vi "Glavna_Programa.vi"() -> ()   [LabVIEW 2021, in "Main.lvlib"]
doc: "Main VI program. \n1. After starting the program, click PowerUP to turn on the calibrator.\n2. The program in Standby can pick the signal values with the use of the keyboard or SetUP mode. \nThe SetUP VI can configure can change the signal type, offset and phase. \n3. Click Operate to go to Operate mode. First 2 Warning message will be shown, then the program will start with Operate mode.\n4. Click Standby to go to standby again, then the program will stop with the DaQ and Operating mode.\n5. Click PowerUP to sotp the program"
uses:
  Main.lvlib
  Tipski Definicii/Kalibrator_Sostojbi.ctl
  Tipski Definicii/QMH_Daq_States.ctl
  Tipski Definicii/error_handl.ctl
  Tipski Definicii/check.ctl
  Tipski Definicii/Keyboard_Sostojbi.ctl
  Tipski Definicii/Signal Values.ctl
  Tipski Definicii/rel_error.ctl
  Tipski Definicii/danger.ctl
  Tipski Definicii/Unit.ctl
  Polymorphic/Init_Main.vi
  <vilib>/Platform/browser.llb/Open URL in Default Browser (path).vi
  Polymorphic/Enq_DaQ_QMH.vi
  Polymorphic/Enq_Calibrator_QMH.vi
  Polymorphic/Prev_Calibrator_QMH.vi
  Polymorphic/DeQ_Calibrator_QMH.vi
  Polymorphic/DaQ_Signal.vi
  Polymorphic/Release_Main.vi
  Signal/Signal.lvlib
  subVIS/Main_Programs_SubVIs.lvlib
  Polymorphic/Queues.lvlib
panel:
  out "AuxA":bool
  out "NormalV":bool
  in  "Knob":dbl(knob) scale=-3.0..3.0 scale format="%#.3g"
  out "Lev_Indikator":string
  out "Desen_Indikator":string
  out "Scope Out":bool
  out "Scope In":bool
  out "AuxAOut":bool
  out "NormalVOut":bool
  in  "V":bool
  in  "Trig":bool
  in  "Tocka":bool
  in  "0":bool
  in  "STBY":bool
  in  "Shift":bool
  in  "SetUP":bool
  in  "Scope":bool
  in  "Save":bool
  in  "Reset":bool
  in  "Power Up":bool
  in  "Plus":bool
  in  "Opr":bool
  in  "Ohm":bool
  in  "NewRef":bool
  in  "Multi":bool
  in  "Meas":bool
  in  "M":bool
  in  "k":bool
  in  "Hz":bool
  in  "F":bool
  in  "Enter":bool
  in  "Earth":bool
  in  "Div":bool
  in  "Conn?":bool
  in  "CE":bool
  in  "C":bool
  in  "Boost":bool
  in  "A":bool
  in  "9":bool
  in  "m":bool
  in  "8":bool
  in  "7":bool
  in  "6":bool
  in  "5":bool
  in  "4":bool
  in  "3":bool
  in  "2":bool
  in  "1":bool
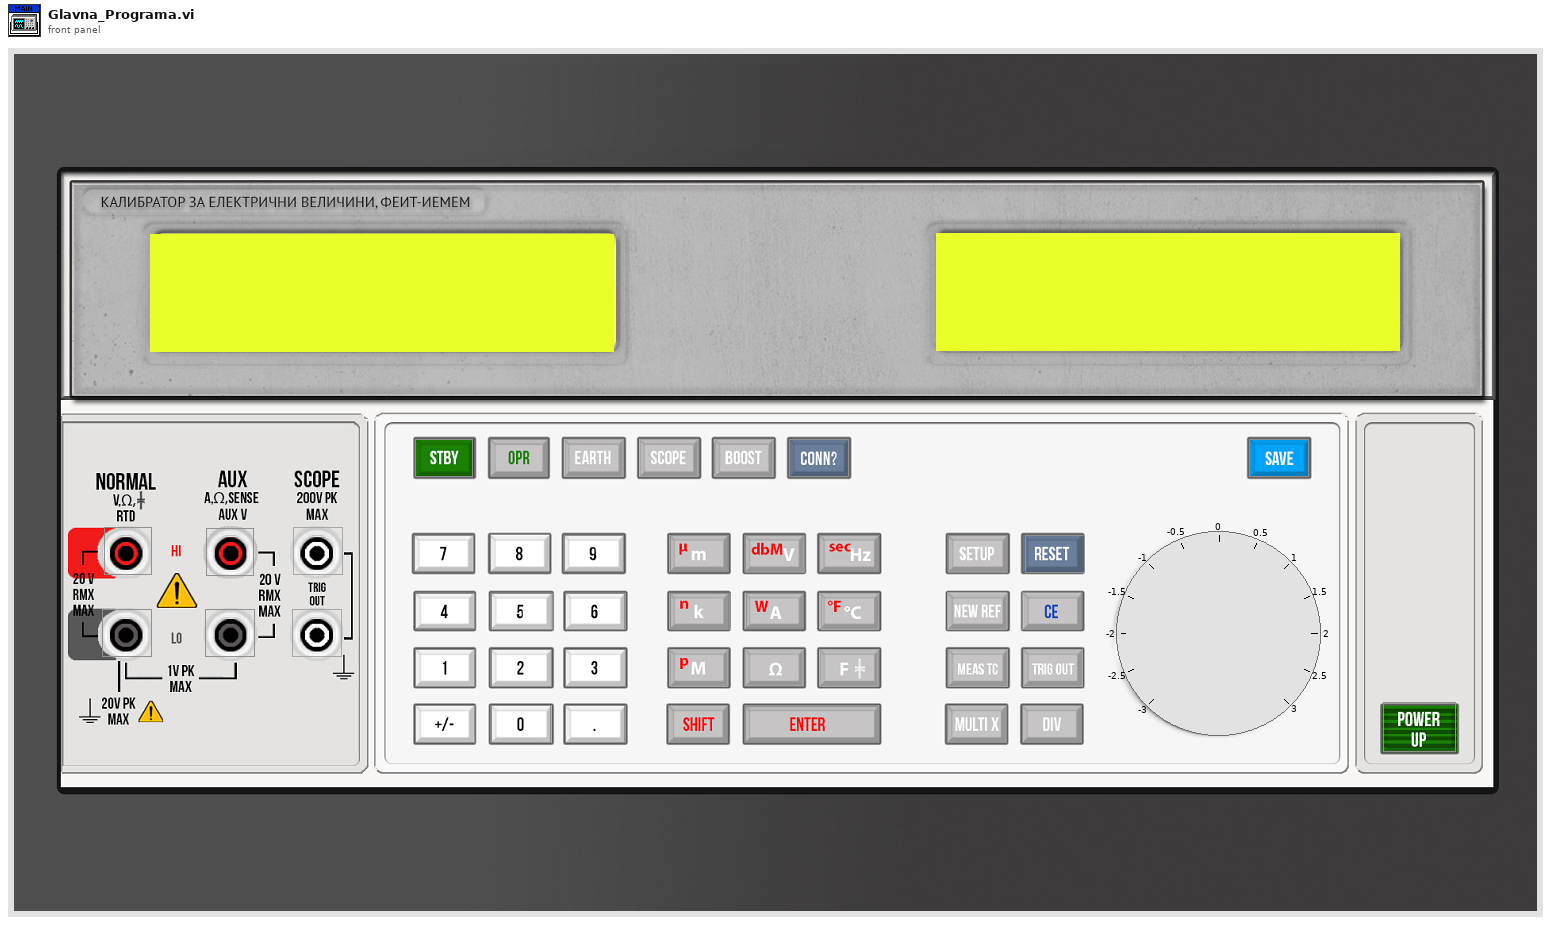
[diagram p1: front panel]
types:
  T1 = cluster{"Calibrator Queue ":refnum<queue>, "ER Refnum":refnum<event-registration>, "User Event in":refnum<user-event>, "QMH Queue ":refnum<queue>, "DaQ":refnum<queue>}
  T2 = typedef "Main_program_queues.ctl" = cluster{"Calibrator QMH":refnum<queue>, "DaQ QMH":refnum<queue>, "DaQ":refnum<queue>, "ER":refnum<event-registration>, "User Event":refnum<user-event>}
  T3 = typedef "error_handl.ctl" = enum16{"Init", "Insert Error 1", "Insert Error 2", "Insert Error 3", "Insert Error 4", "Handle Erros"}
  T4 = enum16{"Init", "Init DaQ", "Start", "Output", "Stop", "Delete", "V/A ?"}
  T5 = typedef "Unit.ctl" = enum16{"Init", "Add", "Read"}
  T6 = typedef "rel_error.ctl" = enum16{"Init", "Add String", "Error", "Get Error and Strings", "Reset"}
  T7 = typedef "danger.ctl" = enum16{"Init", "Check"}
  T8 = typedef "check.ctl" = enum16{"Init", "Add dot", "Add +", "Add Shift", "Check", "Reset", "Reset Shift"}
  T9 = typedef "Signal Values.ctl" = enum16{"Init", "Add V/A string", "Add Hz string", "Get Strings and Values", "Reset", "Add Offset", "Add Waveform", "Add Phase"}
  T10 = typedef "Kalibrator_Sostojbi.ctl" = enum16{"Init", "Idle", "Standby", "Operate ", "End"}
  T11 = typedef "Keyboard_Sostojbi.ctl" = enum16{"Init", "Add Number", "Add Decimal", "Add Unit ", "Clear", "Read", "Enter", "CE", "Add Unit Scale", "Check Unit", "Mul", "Div"}
  T12 = cluster{"Amp String":string, "Amp Value":dbl, "Hz Value Out":dbl, "Waveform Out":enum16{"Sine Wave", "Triangle Wave", "Square Wave", "Sawtooth Wave"}, "Offset Out":dbl, "Phase Out":dbl, "Signal String":string, "Signal":waveform(dbl)}
  T13 = cluster{"Voltage":bool, "Current":bool, "Scope":bool}
  T14 = typedef "QMH_Daq_States.ctl" = enum16{"Idle", "Start DaQ", "DaQ", "Generate Message", "Stop DaQ", "End"}
  T15 = enum32{"Invalid", "Standard", "Closed", "Hidden", "Minimized", "Maximized"}
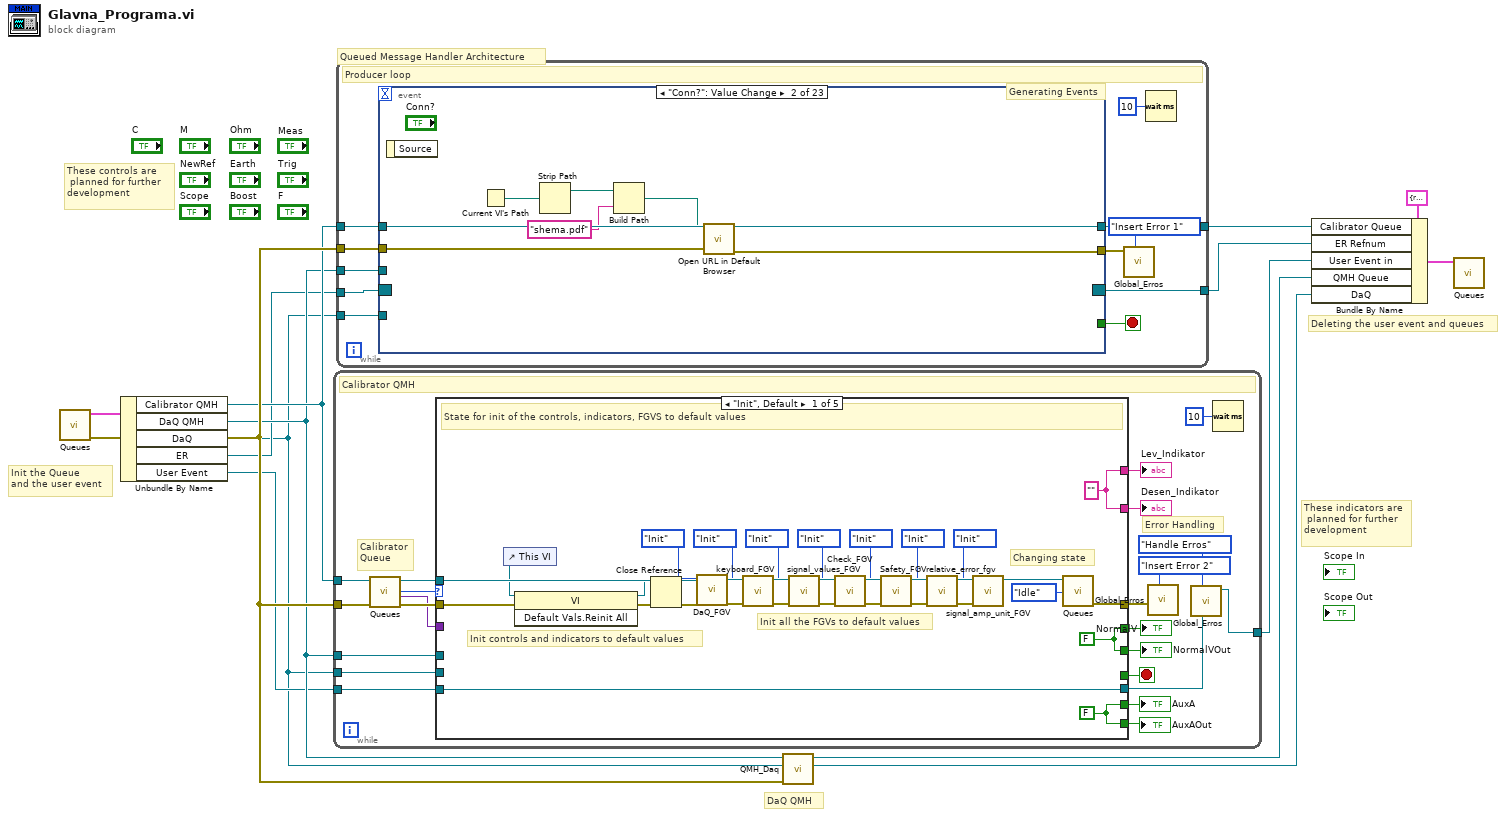
[diagram p0: block diagram]
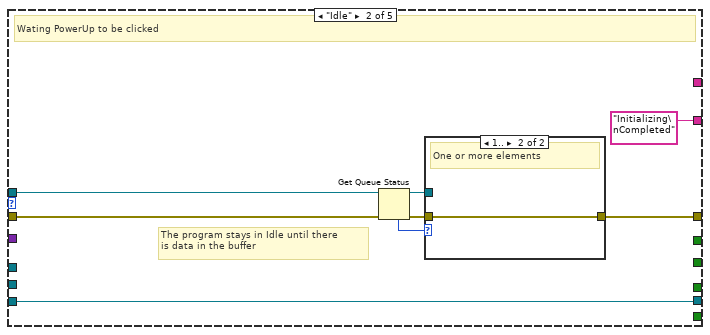
[diagram p2: hidden frame]
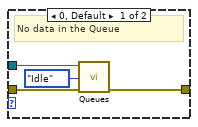
[diagram p3: hidden frame]
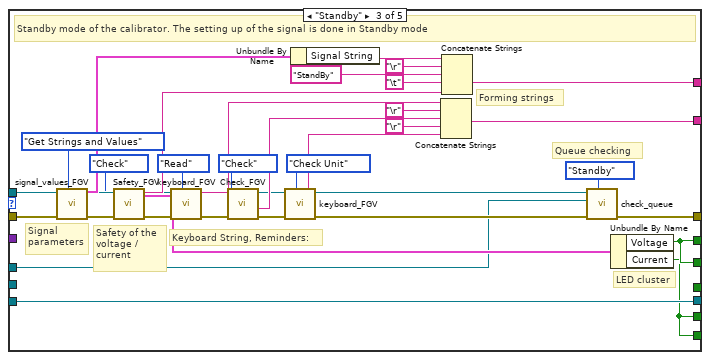
[diagram p4: hidden frame]
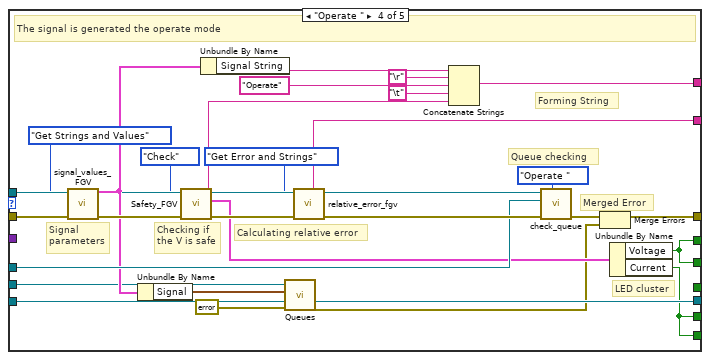
[diagram p5: hidden frame]
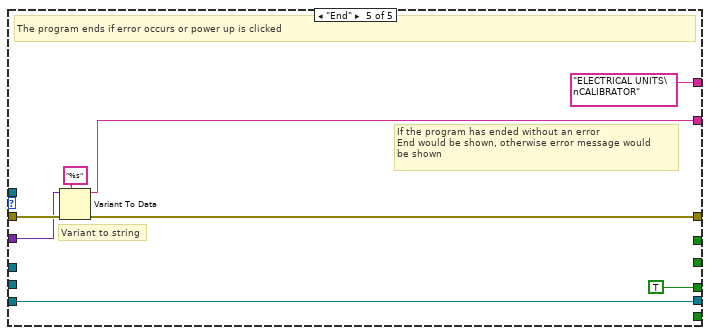
[diagram p6: hidden frame]
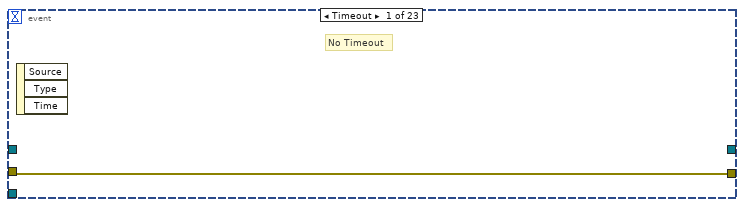
[diagram p7: hidden frame]
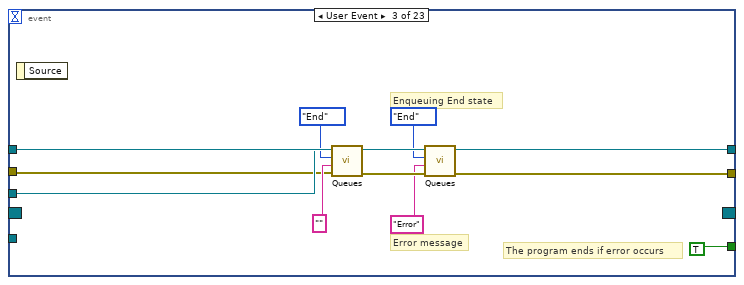
[diagram p8: hidden frame]
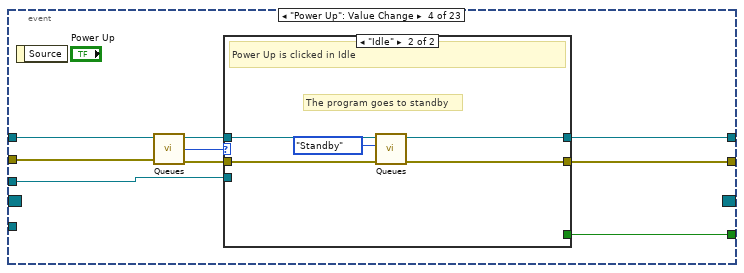
[diagram p9: hidden frame]
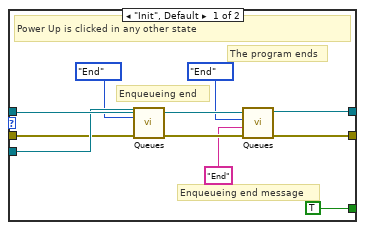
[diagram p10: hidden frame]
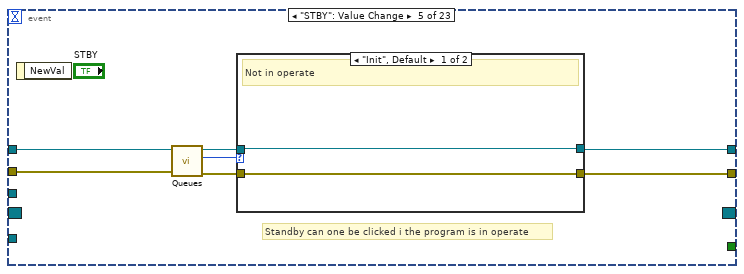
[diagram p11: hidden frame]
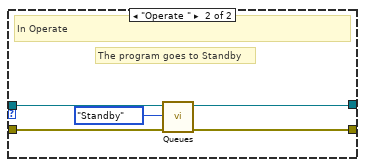
[diagram p12: hidden frame]
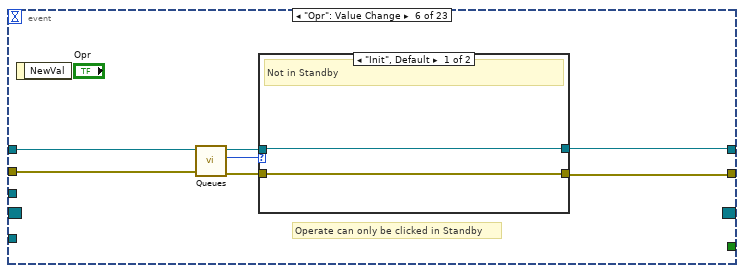
[diagram p13: hidden frame]
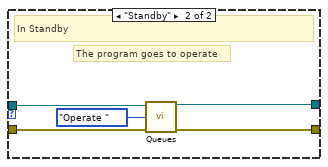
[diagram p14: hidden frame]
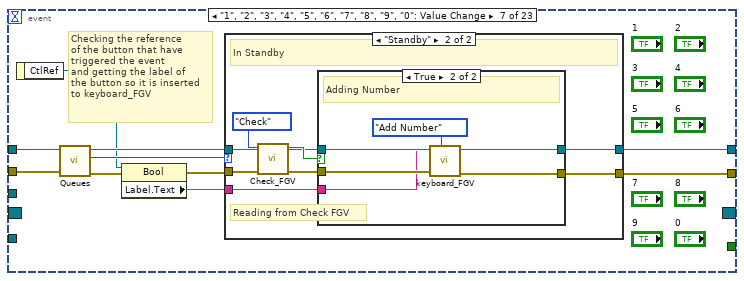
[diagram p15: hidden frame]
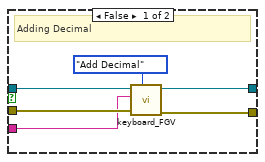
[diagram p17: hidden frame]
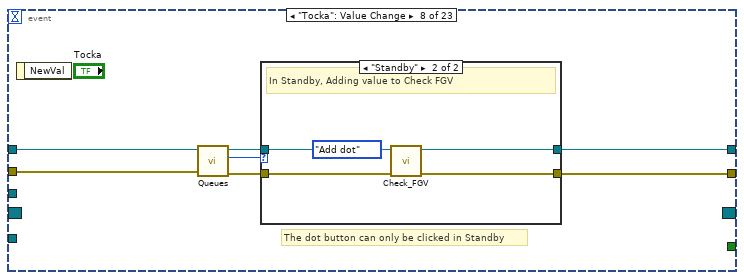
[diagram p18: hidden frame]
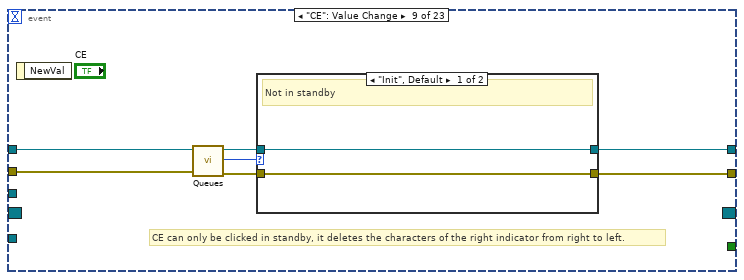
[diagram p20: hidden frame]
diagram:
  # "Init the Queue\nand the user event"
  # "DaQ QMH"
  # "These indicators are\n planned for further \ndevelopment"
  # "These controls are\n planned for further \ndevelopment"
  # "Deleting the user event and queues"
  # "Queued Message Handler Architecture"
  n1 = call-poly "Queues.vi"() -> ("Error Out"=w14:errorcluster, "Queue Cluster"=w13:T2)  [unwired: 10 in]
  n2 = Unbundle By Name(w13) -> ("Calibrator QMH"=w12:refnum<queue>, "DaQ QMH"=w11:refnum<queue>, "DaQ"=w1:refnum<queue>, "ER"=w10:refnum<event-registration>, "User Event"=w9:refnum<user-event>)
  n3 = while {
    tunnel: w9 -> [w33]
    tunnel: [w29] -> w5
    tunnel: w12 -> [w25]
    tunnel: w11 -> [w31]
    tunnel: w1 -> [w32]
    tunnel: w14 -> [w26]
    stop <- w34 stop-if-true
    # "Calibrator\nQueue"
    # "Error Handling"
    # "Calibrator QMH"
    n4 = call-poly "Queues.vi"("Error In"=w26, "Queue In"=w25) -> ("Error Out"=w24:errorcluster, "Message"=w22:variant, "Instruction"=w23:T10, "Queue Out"=w27:refnum<queue>)  [unwired: 6 in]
    n5 = case shown="\"Init\", Default" w23 {
      tunnel: w27 -> [w61 w67 w83 w118 _]
      tunnel: w24 -> [w60 w66 w105 w131 w139]
      tunnel: [w58 "Initializing\nCompleted" ("Desen_Indikator") w99 w126 w136] -> w36
      tunnel: [w58 _ w104 w128 "ELECTRICAL UNITS\nCALIBRATOR" ("Desen_Indikator")] -> w35
      tunnel: [w49 w62 w77 w119 w135] -> w28
      tunnel: [_ _ _ _ TRUE] -> w34
      tunnel: w33 -> [w50 w68 w86 w114 w140]
      tunnel: [w50 w68 w86 w114 w140] -> w30
      tunnel: w31 -> [_ _ w85 w122 _]
      tunnel: w32 -> [_ _ _ w109 _]
      tunnel: w22 -> [_ _ _ _ w137]
      tunnel: [w41 _ w76 w113 _] -> w19
      tunnel: [w41 _ w76 w113 _] -> w18
      tunnel: [w40 _ w75 w111 _] -> w16
      tunnel: [w40 _ w75 w111 _] -> w15
      frame "Init", Default {
        w40 = FALSE ("Current")
        w41 = FALSE ("NormalV")
        w58 = "" ("Desen_Indikator")
        # "Changing state"
        # "Init all the FGVs to default values"
        # "Init controls and indicators to default values"
        # "State for init of the controls, indicators, FGVS to default values"
        n6 = control-ref of="This VI"() -> (w59:refnum<vi>)
        n7 = invoke class="VI" method="Default Vals.Reinit All"(reference=w59, error in=w60) -> (reference out=w56:refnum<vi>, error out=w57:errorcluster)  [unwired: 1 in, 1 out]
        n8 = Close Reference(reference=w56, error in (no error)=w57) -> (error out=w39:errorcluster)
        n9 = call "DaQ_FGV.vi"("Error In"=w39, "Action"=T4."Init") -> ("Error Out"=w38:errorcluster)  [unwired: 9 in]
        n10 = call "keyboard_FGV.vi"("Action"=Keyboard_Sostojbi."Init", "Error In"=w38) -> ("Error Out"=w55:errorcluster)  [unwired: 6 in, 3 out]
        n11 = call "signal_values_FGV.vi"("Action"=Signal_Values."Init", "Error In"=w55) -> ("Error Out"=w54:errorcluster)  [unwired: 12 in, 1 out]
        n12 = call "Check_FGV.vi"("Error In"=w54, "Action"=check."Init") -> ("Error Out"=w53:errorcluster)  [unwired: 5 in, 4 out]
        n13 = call "Safety_FGV.vi"("Error In"=w53, "Action"=danger."Init") -> ("Error Out"=w52:errorcluster)  [unwired: 7 in, 2 out]
        n14 = call "relative_error_fgv.vi"("Error In"=w52, "Action"=rel_error."Init") -> ("Error Out"=w43:errorcluster)  [unwired: 5 in, 4 out]
        n15 = call "signal_amp_unit_FGV.vi"("Error In"=w43, "Action"=Unit."Init") -> ()  [unwired: 7 in, 3 out]
        n16 = call-poly "Queues.vi"("Instruction"=Kalibrator_Sostojbi."Idle", "Queue In"=w61) -> ("Error Out"=w49:errorcluster)  [unwired: 8 in, 1 out]
      }
      frame "Idle" {
        # "The program stays in Idle until there\nis data in the buffer"
        # "Wating PowerUp to be clicked"
        n17 = Get Queue Status(queue=w67, error in (no error)=w66) -> (queue out=w63:refnum<queue>, error out=w64:errorcluster, # elements in queue=w65:i32)  [unwired: 1 in, 5 out]
        n18 = case shown="1.." w65 {
          tunnel: w64 -> [w73 w74]
          tunnel: w63 -> [w72 _]
          tunnel: [w70 w74] -> w62
          frame 0, Default {
            # "No data in the Queue"
            n19 = call-poly "Queues.vi"("Error In"=w73, "Instruction"=Kalibrator_Sostojbi."Idle", "Queue In"=w72) -> ("Error Out"=w70:errorcluster)  [unwired: 7 in, 1 out]
          }
          frame 1.. {
            # "One or more elements"
          }
        }
      }
      frame "Standby" {
        # "LED cluster"
        # "Queue checking"
        # "Forming strings"
        # "Keyboard String, Reminders:"
        # "Safety of the \nvoltage /\ncurrent"
        # "Signal \nparameters"
        # "Standby mode of the calibrator. The setting up of the signal is done in Standby mode"
        n20 = call "signal_values_FGV.vi"("Action"=Signal_Values."Get Strings and Values", "Error In"=w105) -> ("Signal"=w88:T12, "Error Out"=w91:errorcluster)  [unwired: 12 in]
        n21 = call "Safety_FGV.vi"("Error In"=w91, "Action"=danger."Check") -> ("Error Out"=w90:errorcluster, "LED"=w106:T13, "Safetymsg"=w89:string)  [unwired: 7 in]
        n22 = call "keyboard_FGV.vi"("Action"=Keyboard_Sostojbi."Read", "Error In"=w90) -> ("Error Out"=w101:errorcluster, "Indicator Text"=w100:string)  [unwired: 6 in, 2 out]
        n23 = call "Check_FGV.vi"("Error In"=w101, "Action"=check."Check") -> ("Error Out"=w96:errorcluster, "Dot String"=w98:string)  [unwired: 5 in, 3 out]
        n24 = call "keyboard_FGV.vi"("Action"=Keyboard_Sostojbi."Check Unit", "Error In"=w96) -> ("Error Out"=w93:errorcluster, "Unit msg"=w95:string)  [unwired: 6 in, 2 out]
        n25 = Unbundle By Name(w88) -> ("Signal String"=w87:string)
        n26 = Concatenate Strings(w100, "\r", w98, "\r", w95) -> (w99:string)
        n27 = Concatenate Strings(w87, "\r", "StandBy" ("Desen_Indikator"), "\t", w89) -> (w104:string)
        n28 = call "check_queue.vi"("State"=Kalibrator_Sostojbi."Standby", "Error In"=w93, "DaQ QMH"=w85, "Calibrator Queue"=w83) -> ("Error Out"=w77:errorcluster)  [unwired: 7 in]
        n29 = Unbundle By Name(w106) -> ("Voltage"=w76:bool, "Current"=w75:bool)
      }
      frame "Operate " {
        # "Merged Error"
        # "LED cluster"
        # "Forming String"
        # "Queue checking"
        # "Calculating relative error"
        # "Checking if\nthe V is safe"
        # "Signal \nparameters"
        # "The signal is generated the operate mode"
        n30 = call "signal_values_FGV.vi"("Action"=Signal_Values."Get Strings and Values", "Error In"=w131) -> ("Signal"=w121:T12, "Error Out"=w129:errorcluster)  [unwired: 12 in]
        n31 = Unbundle By Name(w121) -> ("Signal"=w108:waveform(dbl))
        n32 = call "Safety_FGV.vi"("Error In"=w129, "Action"=danger."Check") -> ("Error Out"=w127:errorcluster, "LED"=w112:T13, "Safetymsg"=w130:string)  [unwired: 7 in]
        n33 = Unbundle By Name(w121) -> ("Signal String"=w125:string)
        n34 = call-poly "Queues.vi"("Error In"=errorcluster {"status"=FALSE, "code"=0, "source"=""} ("error in (no error)"), "Signal"=w108, "Queue In"=w109) -> ("Error Out"=w107:errorcluster)  [unwired: 7 in, 1 out]
        n35 = call "relative_error_fgv.vi"("Error In"=w127, "Action"=rel_error."Get Error and Strings") -> ("Error Out"=w124:errorcluster, "Indicator String"=w126:string)  [unwired: 5 in, 3 out]
        n36 = Concatenate Strings(w125, "\r", "Operate" ("Desen_Indikator"), "\t", w130) -> (w128:string)
        n37 = call "check_queue.vi"("State"=Kalibrator_Sostojbi."Operate ", "Error In"=w124, "DaQ QMH"=w122, "Calibrator Queue"=w118) -> ("Error Out"=w120:errorcluster)  [unwired: 7 in]
        n38 = Merge Errors(w120, w107) -> (w119:errorcluster)
        n39 = Unbundle By Name(w112) -> ("Voltage"=w113:bool, "Current"=w111:bool)
      }
      frame "End" {
        # "If the program has ended without an error\nEnd would be shown, otherwise error message would\nbe shown"
        # "Variant to string"
        # "The program ends if error occurs or power up is clicked"
        n40 = Variant To Data(error in=w139, type="%s", Variant=w137) -> (data=w136:string, error out=w135:errorcluster)
      }
    }
    "Lev_Indikator" <- w35
    "Desen_Indikator" <- w36
    "NormalVOut" <- w18
    "NormalV" <- w19
    "AuxA" <- w16
    "AuxAOut" <- w15
    n41 = call "Global_Erros.vi"("Action"=error_handl."Insert Error 2", "Error Loop2"=w28) -> ()  [unwired: 9 in, 1 out]
    n42 = call "Global_Erros.vi"("User Event In"=w30, "Action"=error_handl."Handle Erros") -> ("User Event Out"=w29:refnum<user-event>)  [unwired: 9 in]
    n43 = Wait (ms)(milliseconds to wait=u32 10) -> ()  [unwired: 1 out]
  }
  n44 = while {
    tunnel: w12 -> [w153]
    tunnel: w14 -> [w148]
    tunnel: [w152] -> w6
    tunnel: w10 -> [w151]
    tunnel: [w149] -> w7
    tunnel: w11 -> [w147]
    tunnel: w1 -> [w143]
    stop <- w150 stop-if-true
    # "Generating Events"
    # "Producer loop"
    n45 = event shown="[1] \"Conn?\": Value Change" {
      selector: w151 -> [_ _ _ _ _ _ _ _ _ _ _ _ _ _ _ _ _ _ _ _ _ _ _]
      dyn-events: [_ _ _ _ _ _ _ _ _ _ _ _ _ _ _ _ _ _ _ _ _ _ _] -> w152
      timeout: _ -> [_ _ _ _ _ _ _ _ _ _ _ _ _ _ _ _ _ _ _ _ _ _ _]
      tunnel: w153 -> [_ w161 w172 w176 w199 w213 w232 w258 w271 w284 w307 w321 w336 w363 w391 w422 w448 w471 w499 w509 w525 w553 w566]
      tunnel: w148 -> [w154 w160 w162 w177 w201 w215 w233 w259 w272 w285 w309 w322 w335 w364 w392 w424 w449 w473 w500 w513 w526 w554 w567]
      tunnel: [_ w161 w164 w181 w203 w217 w234 w261 w274 w286 w311 w324 w339 w366 w390 w427 w452 w475 w501 w515 w527 w555 w568] -> w149
      tunnel: [w154 w158 w163 w180 w202 w216 w225 w260 w273 w287 w310 w323 w338 w367 w389 w426 w451 w474 w502 w514 w528 w546 w569] -> w144
      tunnel: [_ _ TRUE w179 _ _ _ _ _ _ _ _ _ _ _ _ _ _ _ _ _ _ _] -> w150
      tunnel: w147 -> [_ _ w170 w178 _ _ _ _ _ _ _ _ _ _ _ _ _ _ _ _ _ _ _]
      tunnel: w143 -> [_ _ _ _ _ _ _ _ _ _ _ _ _ _ _ _ _ _ _ _ _ w549 _]
      event Timeout {
        # "No Timeout"
        n46 = event-data() -> ()  [unwired: 1 in, 3 out]
      }
      event "Conn?": Value Change {
        n47 = event-data() -> ()  [unwired: 1 in, 1 out]
        n48 = Current VI's Path() -> (path=w159:path)
        n49 = Strip Path(path=w159) -> (stripped path=w157:path)  [unwired: 1 out]
        n50 = Build Path(base path=w157, name or relative path="shema.pdf") -> (appended path=w155:path)
        n51 = call-poly <vilib>:"Open URL in Default Browser.vi"("error in (no error)"=w160, "path"=w155) -> ("error out"=w158:errorcluster)  [unwired: 4 in, 1 out]
      }
      event User Event {
        # "Enqueuing End state"
        # "Error message"
        # "The program ends if error occurs"
        n52 = event-data() -> ()  [unwired: 1 in, 1 out]
        n53 = call-poly "Queues.vi"("Error In"=w162, "Message"="", "Instruction"=QMH_Daq_States."End", "Queue In"=w170) -> ("Error Out"=w167:errorcluster)  [unwired: 6 in, 1 out]
        n54 = call-poly "Queues.vi"("Error In"=w167, "Message"="Error", "Instruction"=Kalibrator_Sostojbi."End", "Queue In"=w172) -> ("Error Out"=w163:errorcluster, "Queue Out"=w164:refnum<queue>)  [unwired: 6 in]
      }
      event "Power Up": Value Change {
        n55 = event-data() -> ()  [unwired: 1 in, 1 out]
        n56 = call-poly "Queues.vi"("Error In"=w177, "Queue In"=w176) -> ("Error Out"=w173:errorcluster, "Instruction"=w174:T10, "Queue Out"=w175:refnum<queue>)  [unwired: 6 in, 1 out]
        n57 = case shown="\"Idle\"" w174 {
          tunnel: w175 -> [w191 w194]
          tunnel: w173 -> [w182 w196]
          tunnel: [w186 w193] -> w181
          tunnel: [w185 w195] -> w180
          tunnel: [TRUE _] -> w179
          tunnel: w178 -> [w189 _]
          frame "Init", Default {
            # "Enqueueing end"
            # "Enqueueing end message"
            # "The program ends"
            # "Power Up is clicked in any other state"
            n58 = call-poly "Queues.vi"("Error In"=w182, "Instruction"=QMH_Daq_States."End", "Queue In"=w189) -> ("Error Out"=w187:errorcluster)  [unwired: 7 in, 1 out]
            n59 = call-poly "Queues.vi"("Error In"=w187, "Message"="End", "Instruction"=Kalibrator_Sostojbi."End", "Queue In"=w191) -> ("Error Out"=w185:errorcluster, "Queue Out"=w186:refnum<queue>)  [unwired: 6 in]
          }
          frame "Idle" {
            # "The program goes to standby"
            # "Power Up is clicked in Idle"
            n60 = call-poly "Queues.vi"("Error In"=w196, "Instruction"=Kalibrator_Sostojbi."Standby", "Queue In"=w194) -> ("Error Out"=w195:errorcluster, "Queue Out"=w193:refnum<queue>)  [unwired: 7 in]
          }
        }
      }
      event "STBY": Value Change {
        # "Standby can one be clicked i the program is in operate"
        n61 = event-data() -> ()  [unwired: 1 in, 1 out]
        n62 = call-poly "Queues.vi"("Error In"=w201, "Queue In"=w199) -> ("Error Out"=w200:errorcluster, "Instruction"=w197:T10, "Queue Out"=w198:refnum<queue>)  [unwired: 6 in, 1 out]
        n63 = case shown="\"Init\", Default" w197 {
          tunnel: w200 -> [w204 w210]
          tunnel: w198 -> [w205 w208]
          tunnel: [w204 w209] -> w202
          tunnel: [w205 w207] -> w203
          frame "Init", Default {
            # "Not in operate"
          }
          frame "Operate " {
            # "The program goes to Standby"
            # "In Operate"
            n64 = call-poly "Queues.vi"("Error In"=w210, "Instruction"=Kalibrator_Sostojbi."Standby", "Queue In"=w208) -> ("Error Out"=w209:errorcluster, "Queue Out"=w207:refnum<queue>)  [unwired: 7 in]
          }
        }
      }
      event "Opr": Value Change {
        # "Operate can only be clicked in Standby"
        n65 = event-data() -> ()  [unwired: 1 in, 1 out]
        n66 = call-poly "Queues.vi"("Error In"=w215, "Queue In"=w213) -> ("Error Out"=w214:errorcluster, "Instruction"=w211:T10, "Queue Out"=w212:refnum<queue>)  [unwired: 6 in, 1 out]
        n67 = case shown="\"Init\", Default" w211 {
          tunnel: w214 -> [w218 w224]
          tunnel: w212 -> [w219 w222]
          tunnel: [w218 w223] -> w216
          tunnel: [w219 w221] -> w217
          frame "Init", Default {
            # "Not in Standby"
          }
          frame "Standby" {
            # "The program goes to operate"
            # "In Standby"
            n68 = call-poly "Queues.vi"("Error In"=w224, "Instruction"=Kalibrator_Sostojbi."Operate ", "Queue In"=w222) -> ("Error Out"=w223:errorcluster, "Queue Out"=w221:refnum<queue>)  [unwired: 7 in]
          }
        }
      }
      event "1", "2", "3", "4", "5", "6", "7", "8", "9", "0": Value Change {
        # "Checking the reference\nof the button that have \ntriggered the event \nand getting the label of \nthe button so it is inserted \nto keyboard_FGV"
        n69 = event-data() -> ("CtlRef"=w227:refnum<vi>)  [unwired: 1 in]
        n70 = call-poly "Queues.vi"("Error In"=w233, "Queue In"=w232) -> ("Error Out"=w229:errorcluster, "Instruction"=w230:T10, "Queue Out"=w231:refnum<queue>)  [unwired: 6 in, 1 out]
        n71 = property class="Bool"(reference=w227, error in=w229) -> (error out=w228:errorcluster, "Label.Text"=w226:string)  [unwired: 1 out]
        n72 = case shown="\"Standby\"" w230 {
          tunnel: w228 -> [w235 w244]
          tunnel: [w235 w241] -> w225
          tunnel: w231 -> [w236 w240]
          tunnel: [w236 w239] -> w234
          tunnel: w226 -> [_ w238]
          frame "Init", Default {
            # "Not in Standby"
          }
          frame "Standby" {
            # "Reading from Check FGV"
            # "In Standby"
            n73 = call "Check_FGV.vi"("Error In"=w244, "Action"=check."Check") -> ("Error Out"=w242:errorcluster, "Number ?"=w243:bool)  [unwired: 5 in, 3 out]
            n74 = case shown="True" w243 {
              tunnel: w242 -> [w249 w254]
              tunnel: [w248 w252] -> w241
              tunnel: w240 -> [w247 w253]
              tunnel: [w247 w253] -> w239
              tunnel: w238 -> [w245 w250]
              frame False {
                # "Adding Decimal"
                n75 = call "keyboard_FGV.vi"("Action"=Keyboard_Sostojbi."Add Decimal", "Error In"=w249, "Decimal"=w245) -> ("Error Out"=w248:errorcluster)  [unwired: 5 in, 3 out]
              }
              frame True {
                # "Adding Number"
                n76 = call "keyboard_FGV.vi"("Action"=Keyboard_Sostojbi."Add Number", "Error In"=w254, "Number"=w250) -> ("Error Out"=w252:errorcluster)  [unwired: 5 in, 3 out]
              }
            }
          }
        }
      }
      event "Tocka": Value Change {
        # "The dot button can only be clicked in Standby"
        n77 = event-data() -> ()  [unwired: 1 in, 1 out]
        n78 = call-poly "Queues.vi"("Error In"=w259, "Queue In"=w258) -> ("Error Out"=w255:errorcluster, "Instruction"=w256:T10, "Queue Out"=w257:refnum<queue>)  [unwired: 6 in, 1 out]
        n79 = case shown="\"Standby\"" w256 {
          tunnel: w255 -> [w262 w265]
          tunnel: [w263 w267] -> w261
          tunnel: w257 -> [w263 w267]
          tunnel: [w262 w266] -> w260
          frame "Init", Default {
            # "Not in Standby"
          }
          frame "Standby" {
            # "In Standby, Adding value to Check FGV"
            n80 = call "Check_FGV.vi"("Error In"=w265, "Action"=check."Add dot") -> ("Error Out"=w266:errorcluster)  [unwired: 5 in, 4 out]
          }
        }
      }
      event "CE": Value Change {
        # "CE can only be clicked in standby, it deletes the characters of the right indicator from right to left."
        n81 = event-data() -> ()  [unwired: 1 in, 1 out]
        n82 = call-poly "Queues.vi"("Error In"=w272, "Queue In"=w271) -> ("Error Out"=w268:errorcluster, "Instruction"=w269:T10, "Queue Out"=w270:refnum<queue>)  [unwired: 6 in, 1 out]
        n83 = case shown="\"Init\", Default" w269 {
          tunnel: w268 -> [w275 w280]
          tunnel: w270 -> [w276 w279]
          tunnel: [w276 w279] -> w274
          tunnel: [w275 w278] -> w273
          frame "Init", Default {
            # "Not in standby"
          }
          frame "Standby" {
            # "In standby"
            n84 = call "keyboard_FGV.vi"("Action"=Keyboard_Sostojbi."CE", "Error In"=w280) -> ("Error Out"=w278:errorcluster)  [unwired: 6 in, 3 out]
          }
        }
      }
      event "Enter": Value Change {
        # "Enter can only be clicked if the program is in Standby and the electrical unit was picked"
        n85 = event-data() -> ()  [unwired: 1 in, 1 out]
        n86 = call-poly "Queues.vi"("Error In"=w285, "Queue In"=w284) -> ("Error Out"=w282:errorcluster, "Instruction"=w281:T10, "Queue Out"=w283:refnum<queue>)  [unwired: 6 in, 1 out]
        n87 = case shown="\"Standby\"" w281 {
          tunnel: w282 -> [w288 w295]
          tunnel: w283 -> [w289 w292]
          tunnel: [w288 w296] -> w287
          tunnel: [w289 w290] -> w286
          frame "Init", Default {
            # "Not in Standby"
          }
          frame "Standby" {
            # "Checking if unit was entered"
            # "In Standby"
            n88 = call "keyboard_FGV.vi"("Action"=Keyboard_Sostojbi."Check Unit", "Error In"=w295) -> ("Error Out"=w291:errorcluster, "Unit"=w293:bool)  [unwired: 6 in, 2 out]
            n89 = case shown="False" w293 {
              tunnel: [w301 w303] -> w296
              tunnel: [w297 w304] -> w290
              tunnel: w292 -> [w297 w304]
              tunnel: w291 -> [w298 w303]
              frame False {
                # "Unit is entered"
                n90 = call "keyboard_FGV.vi"("Action"=Keyboard_Sostojbi."Enter", "Error In"=w298) -> ("Error Out"=w302:errorcluster)  [unwired: 6 in, 3 out]
                n91 = call "keyboard_FGV.vi"("Action"=Keyboard_Sostojbi."Clear", "Error In"=w302) -> ("Error Out"=w301:errorcluster)  [unwired: 6 in, 3 out]
              }
              frame True {
                # "No unit entered"
              }
            }
          }
        }
      }
      event "Plus": Value Change {
        # "The plus button can only be clicked in Standby, it is used to change the polarity of the voltage"
        n92 = event-data() -> ()  [unwired: 1 in, 1 out]
        n93 = call-poly "Queues.vi"("Error In"=w309, "Queue In"=w307) -> ("Error Out"=w308:errorcluster, "Instruction"=w305:T10, "Queue Out"=w306:refnum<queue>)  [unwired: 6 in, 1 out]
        n94 = case shown="\"Standby\"" w305 {
          tunnel: [w313 w316] -> w311
          tunnel: w306 -> [w313 w316]
          tunnel: w308 -> [w312 w317]
          tunnel: [w312 w315] -> w310
          frame "Init", Default {
            # "Not in Standby"
          }
          frame "Standby" {
            # "Adding value to Check FGV"
            # "In Standby"
            n95 = call "Check_FGV.vi"("Error In"=w317, "Action"=check."Add +") -> ("Error Out"=w315:errorcluster)  [unwired: 5 in, 4 out]
          }
        }
      }
      event "Shift": Value Change {
        # "Shift can only be clicked in Standby. If shift is clicked the usser can pick the \nsecondary options of the units keyboard"
        n96 = event-data() -> ()  [unwired: 1 in, 1 out]
        n97 = call-poly "Queues.vi"("Error In"=w322, "Queue In"=w321) -> ("Error Out"=w319:errorcluster, "Instruction"=w318:T10, "Queue Out"=w320:refnum<queue>)  [unwired: 6 in, 1 out]
        n98 = case shown="\"Standby\"" w318 {
          tunnel: w319 -> [w325 w330]
          tunnel: w320 -> [w326 w329]
          tunnel: [w326 w329] -> w324
          tunnel: [w325 w328] -> w323
          frame "Init", Default {
            # "Not in Standby"
          }
          frame "Standby" {
            # "Adding value to the Shift FGV"
            # "In Standby"
            n99 = call "Check_FGV.vi"("Error In"=w330, "Action"=check."Add Shift") -> ("Error Out"=w328:errorcluster)  [unwired: 5 in, 4 out]
          }
        }
      }
      event "m": Value Change {
        # "Reset shift FGV"
        # "m can only be clicked in standby"
        n100 = event-data() -> ()  [unwired: 1 in, 1 out]
        n101 = call-poly "Queues.vi"("Error In"=w335, "Queue In"=w336) -> ("Error Out"=w332:errorcluster, "Instruction"=w334:T10, "Queue Out"=w333:refnum<queue>)  [unwired: 6 in, 1 out]
        n102 = case shown="\"Standby\"" w334 {
          tunnel: w333 -> [w341 w345]
          tunnel: w332 -> [w340 w348]
          tunnel: [w341 w344] -> w339
          tunnel: [w340 w343] -> w337
          frame "Init", Default {
            # "Not in Standby"
          }
          frame "Standby" {
            # "Checking if shift is clicked before m"
            # "In Standby"
            n103 = call "Check_FGV.vi"("Error In"=w348, "Action"=check."Check") -> ("Error Out"=w346:errorcluster, "Shift ?"=w347:bool)  [unwired: 5 in, 3 out]
            n104 = case shown="False" w347 {
              tunnel: w346 -> [w353 w356]
              tunnel: w345 -> [w350 w355]
              tunnel: [w350 w355] -> w344
              tunnel: [w349 w354] -> w343
              frame False {
                # "No shift clicked"
                n105 = call "keyboard_FGV.vi"("Prefix"="m" ("Unit scale"), "Action"=Keyboard_Sostojbi."Add Unit Scale", "Error In"=w353) -> ("Error Out"=w349:errorcluster)  [unwired: 5 in, 3 out]
              }
              frame True {
                # "Shift clicked"
                n106 = call "keyboard_FGV.vi"("Prefix"="micro" ("Unit scale"), "Action"=Keyboard_Sostojbi."Add Unit Scale", "Error In"=w356) -> ("Error Out"=w354:errorcluster)  [unwired: 5 in, 3 out]
              }
            }
          }
        }
        n107 = call "Check_FGV.vi"("Error In"=w337, "Action"=check."Reset Shift") -> ("Error Out"=w338:errorcluster)  [unwired: 5 in, 4 out]
      }
      event "V": Value Change {
        # "Reseting shift FGV"
        # "V can only be clicked in standby"
        n108 = event-data() -> ()  [unwired: 1 in, 1 out]
        n109 = call-poly "Queues.vi"("Error In"=w364, "Queue In"=w363) -> ("Error Out"=w361:errorcluster, "Instruction"=w360:T10, "Queue Out"=w362:refnum<queue>)  [unwired: 6 in, 1 out]
        n110 = case shown="\"Standby\"" w360 {
          tunnel: w362 -> [w369 w373]
          tunnel: w361 -> [w368 w376]
          tunnel: [w369 w372] -> w366
          tunnel: [w368 w371] -> w365
          frame "Init", Default {
            # "Not in standby"
          }
          frame "Standby" {
            # "Checking if shift is clicked"
            # "In Standby"
            n111 = call "Check_FGV.vi"("Error In"=w376, "Action"=check."Check") -> ("Error Out"=w374:errorcluster, "Shift ?"=w375:bool)  [unwired: 5 in, 3 out]
            n112 = case shown="False" w375 {
              tunnel: w374 -> [w386 w387]
              tunnel: w373 -> [w383 w388]
              tunnel: [w383 w388] -> w372
              tunnel: [w378 w387] -> w371
              frame False {
                # "Shift not clicked"
                n113 = call "keyboard_FGV.vi"("Action"=Keyboard_Sostojbi."Add Unit ", "Error In"=w386, "Unit"="V" ("Unit scale")) -> ("Error Out"=w382:errorcluster)  [unwired: 5 in, 3 out]
                n114 = call "DaQ_FGV.vi"("Error In"=w382, "V/A?"="V", "Action"=T4."V/A ?") -> ("Error Out"=w379:errorcluster)  [unwired: 8 in]
                n115 = call "DaQ_FGV.vi"("Error In"=w379, "Action"=T4."Init DaQ") -> ("Error Out"=w378:errorcluster)  [unwired: 9 in]
              }
              frame True {
                # "Shift clicked"
              }
            }
          }
        }
        n116 = call "Check_FGV.vi"("Error In"=w365, "Action"=check."Reset Shift") -> ("Error Out"=w367:errorcluster)  [unwired: 5 in, 4 out]
      }
      event "A": Value Change {
        # "Reseting shift FGV"
        # "A can only be clicked in standby"
        n117 = event-data() -> ()  [unwired: 1 in, 1 out]
        n118 = call-poly "Queues.vi"("Error In"=w392, "Queue In"=w391) -> ("Error Out"=w395:errorcluster, "Instruction"=w394:T10, "Queue Out"=w396:refnum<queue>)  [unwired: 6 in, 1 out]
        n119 = case shown="\"Standby\"" w394 {
          tunnel: w396 -> [w399 w403]
          tunnel: w395 -> [w398 w406]
          tunnel: [w399 w402] -> w390
          tunnel: [w398 w401] -> w397
          frame "Init", Default {
            # "Not in standby"
          }
          frame "Standby" {
            # "Checking if shift was clicked"
            # "In Standby"
            n120 = call "Check_FGV.vi"("Error In"=w406, "Action"=check."Check") -> ("Error Out"=w404:errorcluster, "Shift ?"=w405:bool)  [unwired: 5 in, 3 out]
            n121 = case shown="False" w405 {
              tunnel: w404 -> [w416 w417]
              tunnel: w403 -> [w413 w418]
              tunnel: [w413 w418] -> w402
              tunnel: [w408 w417] -> w401
              frame False {
                # "Shift was not clicked"
                n122 = call "keyboard_FGV.vi"("Action"=Keyboard_Sostojbi."Add Unit ", "Error In"=w416, "Unit"="A" ("Unit scale")) -> ("Error Out"=w412:errorcluster)  [unwired: 5 in, 3 out]
                n123 = call "DaQ_FGV.vi"("Error In"=w412, "V/A?"="A", "Action"=T4."V/A ?") -> ("Error Out"=w409:errorcluster)  [unwired: 8 in]
                n124 = call "DaQ_FGV.vi"("Error In"=w409, "Action"=T4."Init DaQ") -> ("Error Out"=w408:errorcluster)  [unwired: 9 in]
              }
              frame True {
                # "Shift was clicked"
              }
            }
          }
        }
        n125 = call "Check_FGV.vi"("Error In"=w397, "Action"=check."Reset Shift") -> ("Error Out"=w389:errorcluster)  [unwired: 5 in, 4 out]
      }
      event "Hz": Value Change {
        # "Reseting shift FGV"
        # "Hz can only be clicked in Standby"
        n126 = event-data() -> ()  [unwired: 1 in, 1 out]
        n127 = call-poly "Queues.vi"("Error In"=w424, "Queue In"=w422) -> ("Error Out"=w423:errorcluster, "Instruction"=w420:T10, "Queue Out"=w421:refnum<queue>)  [unwired: 6 in, 1 out]
        n128 = case shown="\"Standby\"" w420 {
          tunnel: w421 -> [w429 w433]
          tunnel: w423 -> [w428 w436]
          tunnel: [w429 w432] -> w427
          tunnel: [w428 w431] -> w425
          frame "Init", Default {
            # "Not in standby"
          }
          frame "Standby" {
            # "Checking if shift is clicked"
            # "In standby"
            n129 = call "Check_FGV.vi"("Error In"=w436, "Action"=check."Check") -> ("Error Out"=w434:errorcluster, "Shift ?"=w435:bool)  [unwired: 5 in, 3 out]
            n130 = case shown="False" w435 {
              tunnel: w434 -> [w441 w442]
              tunnel: w433 -> [w439 w443]
              tunnel: [w439 w443] -> w432
              tunnel: [w438 w442] -> w431
              frame False {
                # "Shift was not clicked"
                n131 = call "keyboard_FGV.vi"("Action"=Keyboard_Sostojbi."Add Unit ", "Error In"=w441, "Unit"="Hz" ("Unit scale")) -> ("Error Out"=w438:errorcluster)  [unwired: 5 in, 3 out]
              }
              frame True {
                # "Shift clicked"
              }
            }
          }
        }
        n132 = call "Check_FGV.vi"("Error In"=w425, "Action"=check."Reset Shift") -> ("Error Out"=w426:errorcluster)  [unwired: 5 in, 4 out]
      }
      event "k": Value Change {
        # "Reseting shfit FGV"
        # "k can only be clicked in standby"
        n133 = event-data() -> ()  [unwired: 1 in, 1 out]
        n134 = call-poly "Queues.vi"("Error In"=w449, "Queue In"=w448) -> ("Error Out"=w446:errorcluster, "Instruction"=w445:T10, "Queue Out"=w447:refnum<queue>)  [unwired: 6 in, 1 out]
        n135 = case shown="\"Standby\"" w445 {
          tunnel: w447 -> [w454 w458]
          tunnel: w446 -> [w453 w461]
          tunnel: [w454 w457] -> w452
          tunnel: [w453 w456] -> w450
          frame "Init", Default {
            # "Not in standby"
          }
          frame "Standby" {
            # "Checking if shift was clicked"
            # "In standby"
            n136 = call "Check_FGV.vi"("Error In"=w461, "Action"=check."Check") -> ("Error Out"=w459:errorcluster, "Shift ?"=w460:bool)  [unwired: 5 in, 3 out]
            n137 = case shown="False" w460 {
              tunnel: w459 -> [w464 w467]
              tunnel: w458 -> [w463 w468]
              tunnel: [w463 w468] -> w457
              tunnel: [w462 w467] -> w456
              frame False {
                # "Shift Not clicked"
                n138 = call "keyboard_FGV.vi"("Prefix"="k" ("Unit scale"), "Action"=Keyboard_Sostojbi."Add Unit Scale", "Error In"=w464) -> ("Error Out"=w462:errorcluster)  [unwired: 5 in, 3 out]
              }
              frame True {
                # "Shift clicked"
              }
            }
          }
        }
        n139 = call "Check_FGV.vi"("Error In"=w450, "Action"=check."Reset Shift") -> ("Error Out"=w451:errorcluster)  [unwired: 5 in, 4 out]
      }
      event "Reset": Value Change {
        # "Reset can only be clicked if the program is not in idle"
        n140 = event-data() -> ()  [unwired: 1 in, 1 out]
        n141 = call-poly "Queues.vi"("Error In"=w473, "Queue In"=w471) -> ("Error Out"=w472:errorcluster, "Instruction"=w469:T10, "Queue Out"=w470:refnum<queue>)  [unwired: 6 in, 1 out]
        n142 = case shown="\"Idle\"" w469 {
          tunnel: [w482 w495] -> w475
          tunnel: w470 -> [w486 w495]
          tunnel: w472 -> [w485 w494]
          tunnel: [w481 w494] -> w474
          frame "Init", Default {
            # "Reseting keyboard FGV, and signal values FGV"
            # "Not in Idle"
            n143 = call "keyboard_FGV.vi"("Action"=Keyboard_Sostojbi."Clear", "Error In"=w485) -> ("Error Out"=w484:errorcluster)  [unwired: 6 in, 3 out]
            n144 = call "signal_values_FGV.vi"("Action"=Signal_Values."Reset", "Error In"=w484) -> ("Error Out"=w480:errorcluster)  [unwired: 12 in, 1 out]
            n145 = call-poly "Queues.vi"("Error In"=w480, "Queue In"=w486) -> ("Error Out"=w478:errorcluster, "Instruction"=w477:T10, "Queue Out"=w479:refnum<queue>)  [unwired: 6 in, 1 out]
            n146 = case shown="\"Operate \", Default" w477 {
              tunnel: w478 -> [w491 w493]
              tunnel: w479 -> [w489 w492]
              tunnel: [w488 w492] -> w482
              tunnel: [w490 w493] -> w481
              frame "Operate ", Default {
                # "The program goes\nto Stadnby"
                # "Clicked in Operate"
                n147 = call-poly "Queues.vi"("Error In"=w491, "Instruction"=Kalibrator_Sostojbi."Standby", "Queue In"=w489) -> ("Error Out"=w490:errorcluster, "Queue Out"=w488:refnum<queue>)  [unwired: 7 in]
              }
              frame "Standby" {
                # "The program stays in\nstandby"
                # "Reset clicked in standby"
              }
            }
          }
          frame "Idle" {
            # "In idle"
          }
        }
      }
      event "Multi": Value Change {
        # "Multi, can only be clicekd in Standby, and is used to \nmultiply the keyboard value by 10."
        n148 = event-data() -> ()  [unwired: 1 in, 1 out]
        n149 = call-poly "Queues.vi"("Error In"=w500, "Queue In"=w499) -> ("Error Out"=w497:errorcluster, "Instruction"=w496:T10, "Queue Out"=w498:refnum<queue>)  [unwired: 6 in, 1 out]
        n150 = case shown="\"Standby\"" w496 {
          tunnel: [w503 w505] -> w502
          tunnel: w498 -> [w504 w507]
          tunnel: [w504 w507] -> w501
          tunnel: w497 -> [w503 w506]
          frame "Init", Default {
            # "Not in standby"
          }
          frame "Standby" {
            # "In standby"
            n151 = call "keyboard_FGV.vi"("Action"=Keyboard_Sostojbi."Mul", "Error In"=w506) -> ("Error Out"=w505:errorcluster)  [unwired: 6 in, 3 out]
          }
        }
      }
      event "Div": Value Change {
        # "Div, can only be clicekd in Standby, and is used to \ndivide the keyboard value by 10."
        n152 = event-data() -> ()  [unwired: 1 in, 1 out]
        n153 = call-poly "Queues.vi"("Error In"=w513, "Queue In"=w509) -> ("Error Out"=w512:errorcluster, "Instruction"=w511:T10, "Queue Out"=w510:refnum<queue>)  [unwired: 6 in, 1 out]
        n154 = case shown="\"Standby\"" w511 {
          tunnel: [w516 w520] -> w514
          tunnel: w512 -> [w516 w519]
          tunnel: w510 -> [w517 w518]
          tunnel: [w517 w518] -> w515
          frame "Init", Default {
            # "Not in Standby"
          }
          frame "Standby" {
            # "Standby"
            n155 = call "keyboard_FGV.vi"("Action"=Keyboard_Sostojbi."Div", "Error In"=w519) -> ("Error Out"=w520:errorcluster)  [unwired: 6 in, 3 out]
          }
        }
      }
      event "SetUP": Value Change {
        # "Opening  \nMaximized\nFront Panel"
        # "Minimazing the main VI"
        # "SetUp can only be clicked if the program is not in idle\nThen the SetUP VI will be opened"
        n156 = event-data() -> ()  [unwired: 1 in, 1 out]
        n157 = call-poly "Queues.vi"("Error In"=w526, "Queue In"=w525) -> ("Error Out"=w523:errorcluster, "Instruction"=w522:T10, "Queue Out"=w524:refnum<queue>)  [unwired: 6 in, 1 out]
        n158 = case shown="\"Idle\", Default" w522 {
          tunnel: w523 -> [w533 w543]
          tunnel: [w530 w543] -> w528
          tunnel: w524 -> [w538 w544]
          tunnel: [w538 w544] -> w527
          frame "Standby" {
            # "Run Vi"
            # "SetUP reference"
            # "Not in Idle"
            n159 = control-ref of="This VI"() -> (w536:refnum<vi>)
            n160 = property class="VI"(reference=w536, error in=w533, "FP.State"=T15."Minimized" ("Front Panel Window:State")) -> (reference out=w537:refnum<vi>, error out=w535:errorcluster)
            n161 = Close Reference(reference=w537, error in (no error)=w535) -> (error out=w532:errorcluster)
            n162 = vi-ref "Setup.vi"() -> (w542:refnum<vi>)
            n163 = invoke class="VI" method="FP.Open"(reference=w542, error in=w532, "Activate"=TRUE ("Activate?"), "State"=T15."Maximized") -> (reference out=w540:refnum<vi>, error out=w539:errorcluster)  [unwired: 1 in, 3 out]
            n164 = invoke class="VI" method="Run VI"(reference=w540, error in=w539, "Auto Dispose Ref"=TRUE ("Auto Dispose Reference")) -> (error out=w530:errorcluster)  [unwired: 2 in, 4 out]
          }
          frame "Idle", Default {
            # "In Idle"
          }
        }
      }
      event "Knob": Value Change {
        # "The DAQ queue is released so the new \nvalue is sent"
        n165 = event-data() -> ()  [unwired: 1 in, 1 out]
        n166 = call-poly "Queues.vi"("Error In"=w554, "Queue In"=w553) -> ("Error Out"=w551:errorcluster, "Instruction"=w550:T10, "Queue Out"=w552:refnum<queue>)  [unwired: 6 in, 1 out]
        n167 = case shown="\"Operate \"" w550 {
          tunnel: [w556 w561] -> w547
          tunnel: w552 -> [w557 w560]
          tunnel: [w557 w560] -> w555
          tunnel: w551 -> [w556 w559]
          frame "Init", Default {
            # "Not In operate"
          }
          frame "Operate " {
            # "In Operate"
            n168 = call "relative_error_fgv.vi"("Error In"=w559, "Knob"="Knob", "Action"=rel_error."Error") -> ("Error Out"=w561:errorcluster)  [unwired: 4 in, 4 out]
          }
        }
        n169 = Flush Queue(queue=w549, error in (no error)=errorcluster {"status"=FALSE, "code"=0, "source"=""}) -> (error out=w545:errorcluster)  [unwired: 2 out]
        n170 = Merge Errors(w547, w545) -> (w546:errorcluster)
      }
      event "Save": Value Change {
        # "Save can only be clicked in operate"
        n171 = event-data() -> ()  [unwired: 1 in, 1 out]
        n172 = call-poly "Queues.vi"("Error In"=w567, "Queue In"=w566) -> ("Error Out"=w564:errorcluster, "Instruction"=w563:T10, "Queue Out"=w565:refnum<queue>)  [unwired: 6 in, 1 out]
        n173 = case shown="\"Operate \"" w563 {
          tunnel: w564 -> [w570 w577]
          tunnel: [w570 w573] -> w569
          tunnel: w565 -> [w571 w575]
          tunnel: [w571 w575] -> w568
          frame "Init", Default {
            # "Not in operate"
          }
          frame "Operate " {
            # "Opening  \nMaximized\nFront Panel"
            # "Save reference"
            # "In operate"
            n174 = control-ref of="This VI"() -> (w580:refnum<vi>)
            n175 = property class="VI"(reference=w580, error in=w577, "FP.State"=T15."Minimized" ("Front Panel Window:State")) -> (reference out=w581:refnum<vi>, error out=w579:errorcluster)
            n176 = Close Reference(reference=w581, error in (no error)=w579) -> (error out=w576:errorcluster)
            n177 = vi-ref "Save.vi"() -> (w585:refnum<vi>)
            n178 = invoke class="VI" method="FP.Open"(reference=w585, error in=w576, "Activate"=TRUE ("Activate?"), "State"=T15."Maximized") -> (reference out=w583:refnum<vi>, error out=w582:errorcluster)  [unwired: 1 in, 3 out]
            n179 = invoke class="VI" method="Run VI"(reference=w583, error in=w582, "Auto Dispose Ref"=TRUE ("Auto Dispose Reference")) -> (error out=w573:errorcluster)  [unwired: 2 in, 4 out]
          }
        }
      }
    }
    n180 = call "Global_Erros.vi"("Action"=error_handl."Insert Error 1", "Error Loop 1"=w144) -> ()  [unwired: 9 in, 1 out]
    n181 = Wait (ms)(milliseconds to wait=u32 10) -> ()  [unwired: 1 out]
  }
  n182 = call "QMH_Daq.vi"("Error In"=w14, "DaQ Queue In"=w1, "QMH Queue"=w11) -> ("DaQ Queue Out"=w3:refnum<queue>, "QMH Queue Out"=w4:refnum<queue>)  [unwired: 7 in]
  n183 = Bundle By Name(cluster=T1 {"Calibrator Queue "=refnum, "ER Refnum"=refnum, "User Event in"=refnum, "QMH Queue "=refnum, "DaQ"=refnum} ("Input Cluster"), "Calibrator Queue"=w7, "ER Refnum"=w6, "User Event in"=w5, "QMH Queue"=w4, "DaQ"=w3) -> (w2:T1)
  n184 = call-poly "Queues.vi"("Queues"=w2) -> ()  [unwired: 11 in]
